vi "Get Mouse Location (Connections).vi"(10 "Event Coord":T1, 11 "Connections Reference":refnum<vi>) -> (0 "in data range":bool, 1 "Element Reference":refnum<vi>, 2 "Type":enum16{"Source", "Destination", "Neither"}(ring), 3 "Array Index":i32)   [LabVIEW 2020, in "Routing and Faulting System Explorer.lvlib"]
uses:
  Routing and Faulting System Explorer.lvlib
  <vilib>/Utility/miscctls.llb/LVPoint32TypeDef.ctl
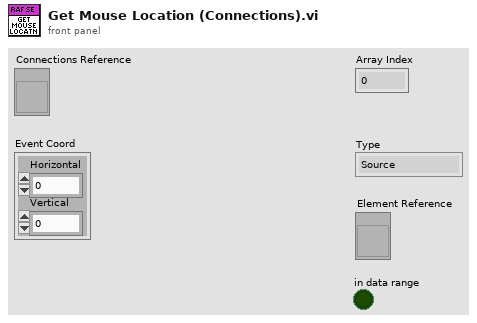
[diagram p1: front panel]
types:
  T1 = typedef "LVPoint32TypeDef.ctl" = cluster{"Horizontal":i32, "Vertical":i32}
  T2 = typedef "Routing and Faulting System Explorer.lvlib/Connection Row.ctl" = cluster{"Source":string, "Destination":string, "Edit":bool, "Remove":bool}
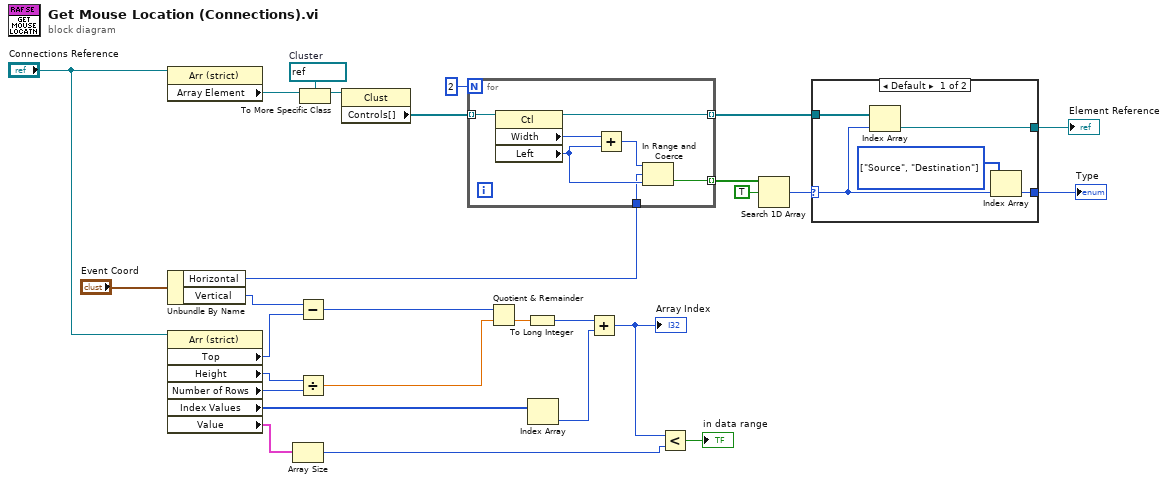
[diagram p0: block diagram]
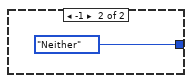
[diagram p2: hidden frame]
diagram:
  w28 = refnum<vi> refnum  # Cluster
  n1 = property on="Property Node" class="Arr (strict)"(reference="Connections Reference") -> ("Array Element"=w26:refnum<vi>)  [unwired: 1 in, 2 out]
  n2 = Unbundle By Name("Event Coord") -> ("Horizontal"=w11:i32, "Vertical"=w17:i32)
  n3 = property on="Property Node" class="Arr (strict)"(reference="Connections Reference") -> ("Top"=w18:i32, "Height"=w19:u32, "Number of Rows"=w21:u32, "Index Values"=w15:u32[], "Value"=w5:T2[])  [unwired: 1 in, 2 out]
  n4 = Array Size(array=w5) -> (size(s)=w3:i32)
  n5 = Subtract(x=w17, y=w18) -> (x-y=w25:i32)
  n6 = Divide(x=w19, y=w21) -> (x/y=w24:dbl)
  n7 = To More Specific Class(target class=w28, reference=w26) -> (specific class reference=w27:refnum<vi>)  [unwired: 1 in, 1 out]
  n8 = property class="Clust"(reference=w27) -> ("Controls[]"=w13:refnum<vi>[])  [unwired: 1 in, 2 out]
  n9 = for {
    N: 2 -> [_]
    tunnel: [w33] -> w10 mode=indexing
    tunnel: w13 -> [w31] mode=indexing
    tunnel: w11 -> [w30]
    tunnel: [w29] -> w7 mode=indexing
    n10 = property on="Property Node" class="Ctl"(reference=w31) -> (reference out=w29:refnum<vi>, "Width"=w32:u32, "Left"=w34:i32)  [unwired: 1 in, 1 out]
    n11 = Add(x=w32, y=w34) -> (x+y=w35:u32)
    n12 = In Range and Coerce(upper limit=w35, x=w30, lower limit=w34) -> (In Range?=w33:bool)  [unwired: 1 out]
  }
  n13 = Quotient & Remainder(x=w25, y=w24) -> (floor(x/y)=w23:dbl)  [unwired: 1 out]
  n14 = To Long Integer(number=w23) -> (32bit integer=w22:i32)
  n15 = Index Array(array=w15) -> (element=w14:u32)  [unwired: 1 in]
  n16 = Add(x=w22, y=w14) -> (x+y=w4:u32)
  "Array Index" <- w4
  n17 = Less?(x=w4, y=w3) -> (x < y?=→"in data range":bool)
  n18 = Search 1D Array(1D array=w10, element=TRUE) -> (index of element=w8:i32)  [unwired: 1 in]
  n19 = case shown="Default" w8 {
    selector: w8 -> [w36 _]
    tunnel: w7 -> [w40 _]
    tunnel: [w39 _] -> w6
    tunnel: [w37 enum16{"Source", "Destination", "Neither"}."Neither" ("type")] -> w2
    frame Default {
      w38 = enum16{"Source", "Destination", "Neither"}[] [enum."Source", enum."Destination"] items=["Source", "Destination", "Neither"]
      n20 = Index Array(array=w40, index=w36) -> (element=w39:refnum<vi>)
      n21 = Index Array(array=w38, index=w36) -> (element=w37:enum16{"Source", "Destination", "Neither"})
    }
    frame -1 {
    }
  }
  "Element Reference" <- w6
  "Type" <- w2
